vi "Destroy Broadcast Events.vi"(8 "error in":errorcluster) -> (0 "error out":errorcluster)   [LabVIEW 2026, in "FT-818 CW Key Control.lvlib"]
doc: "Destroy the broadcast events, even if there is an incoming error.\n\n<b>NOTE</b>: The contents of this VI are automatically generated and modified by the <b>Tools > DQMH Consortium > DQMH</b> utilities. Consider using those utilities instead of making your own modifications to this VI.\n_____\nBased on DQMH Dev Tools: Project Template 7.1.2.1547."
uses:
  FT-818 CW Key Control.lvlib
panel:
  # "NOTE: The contents of this VI are automatically generated and modified by the Tools > DQMH Consortium > DQMH utilities. Consider using those utilities instead of making your own modifications to this VI."
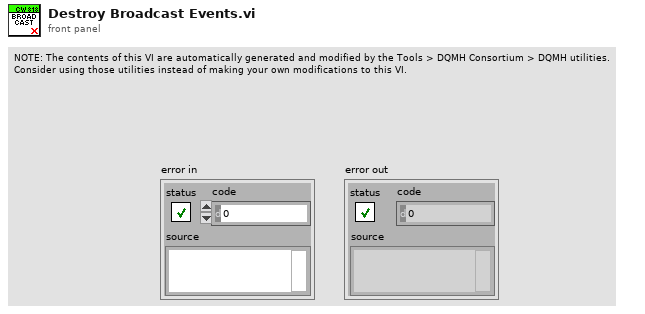
[diagram p1: front panel]
types:
  T1 = typedef "FT-818 CW Key Control.lvlib/Broadcast Events--cluster.ctl" = cluster{"Module Did Init":refnum<user-event>, "Status Updated":refnum<user-event>, "Error Reported":refnum<user-event>, "Module Did Stop":refnum<user-event>, "Update Module Execution Status":refnum<user-event>}
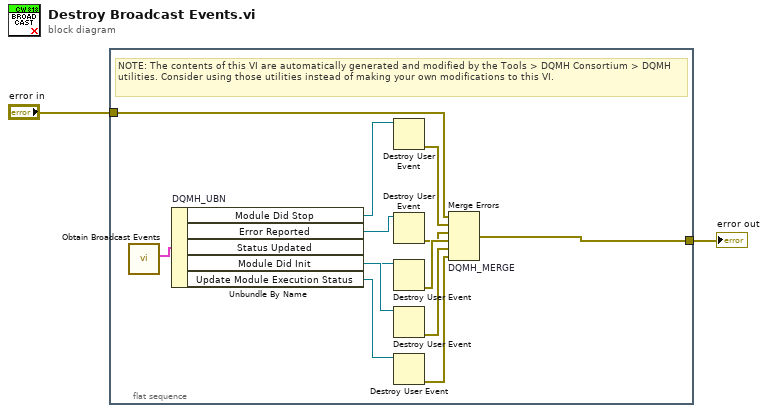
[diagram p0: block diagram]
diagram:
  n1 = flat-sequence {
    tunnel: [w14] -> w2
    tunnel: "error in" -> [w5]
    frame #0 {
      # "NOTE: The contents of this VI are automatically generated and modified by the Tools > DQMH Consortium > DQMH utilities. Consider using those utilities instead of making your own modifications to this VI."
      n2 = call "Obtain Broadcast Events.vi"() -> ("FT-818 CW Key Control Broadcast Events"=w13:T1)  [unwired: 10 in, 1 out]
      n3 = Unbundle By Name "DQMH_UBN"(w13) -> ("Module Did Stop"=w6:refnum<user-event>, "Error Reported"=w8:refnum<user-event>, "Status Updated"=w11:refnum<user-event>, "Module Did Init"=w12:refnum<user-event>, "Update Module Execution Status"=w3:refnum<user-event>)
      n4 = Destroy User Event(user event=w6) -> (error out=w7:errorcluster)  [unwired: 1 in]
      n5 = Destroy User Event(user event=w8) -> (error out=w9:errorcluster)  [unwired: 1 in]
      n6 = Destroy User Event(user event=w11) -> (error out=w10:errorcluster)  [unwired: 1 in]
      n7 = Destroy User Event(user event=w12) -> (error out=w15:errorcluster)  [unwired: 1 in]
      n8 = Destroy User Event(user event=w3) -> (error out=w4:errorcluster)  [unwired: 1 in]
      n9 = Merge Errors "DQMH_MERGE"(w5, w7, w9, w10, w15, w4) -> (w14:errorcluster)
    }
  }
  "error out" <- w2
